vi "Write Profiles.vi"(8 "error in (no error)":errorcluster, 10 "Profiles":T1, 11 "Realsense Cam in":refnum<class "Realsense Cam.lvclass">) -> (0 "error out":errorcluster, 3 "Realsense Cam out":refnum<class "Realsense Cam.lvclass">)   [LabVIEW 2018, in "Realsense Cam.lvclass"]
uses:
  Realsense Cam.lvclass
  Private/Cam Profiles STYP.ctl
  Private/Stream STYP.ctl
  Private/Stream Frame Data STYP.ctl
  Realsense Cam.lvclass/Realsense Cam.ctl
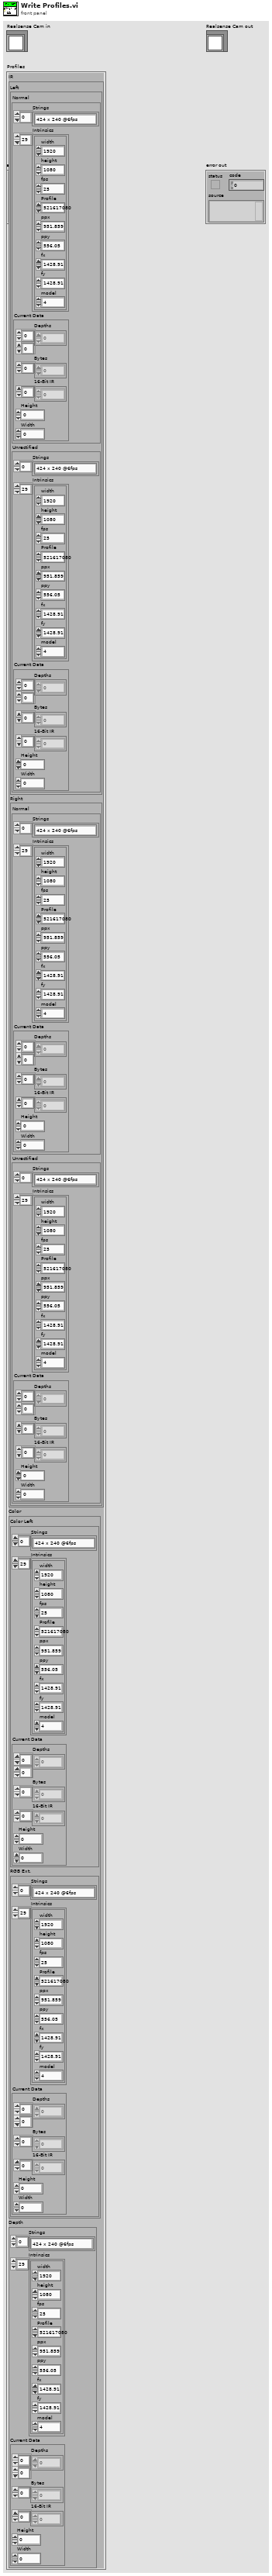
[diagram p1: front panel]
types:
  T1 = typedef "Realsense Cam.lvclass/Cam Profiles STYP.ctl" = cluster{"IR":cluster{"Left":cluster{"Normal":T2, "Unrectified":T2}, "Right":cluster{"Normal":T2, "Unrectified":T2}}, "Color":cluster{"Color Left":T2, "RGB Ext.":T2}, "Depth":T2}
  T2 = typedef "Realsense Cam.lvclass/Stream STYP.ctl" = cluster{"Strings":string[], "Intrinsics":cluster{"width":i32, "height":i32, "fps":i32, "Profile":u64, "ppx":sgl, "ppy":sgl, "fx":sgl, "fy":sgl, "model":u32}[], "Current Data":T3}
  T3 = typedef "Realsense Cam.lvclass/Stream Frame Data STYP.ctl" = cluster{"Depths":sgl[][], "Bytes":u8[], "16-Bit IR":u16[], "Height":i32, "Width":i32}
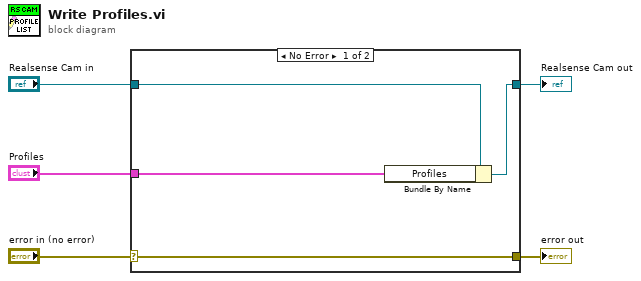
[diagram p0: block diagram]
diagram:
  n1 = case shown="No Error" "error in (no error)" {
    selector: "error in (no error)" -> [w9 w10]
    tunnel: [w9 w10] -> w4
    tunnel: [w7 w11] -> w2
    tunnel: "Realsense Cam in" -> [w8 w11]
    tunnel: "Profiles" -> [w6 _]
    frame No Error {
      n2 = Bundle By Name(cluster=w8, "Profiles"=w6) -> (w7:refnum<class "Realsense Cam.lvclass">)
    }
    frame Error {
    }
  }
  "error out" <- w4
  "Realsense Cam out" <- w2
